vi "MEMR-Read Raw Data File (single traces).vi"(0 "Path":path=path "D:/Data/MEMR/Ken/SFMH41-MEMR-1.txt", 7 "index":i32, 9 "length":i32, 11 "error in":errorcluster) -> (8 "Array":dbl[][](array[numeric]), 15 "error out":errorcluster)   [LabVIEW 2020]
uses:
  PXI DAQ VIs/Utility VIs/Array Dimensions (2D).vi
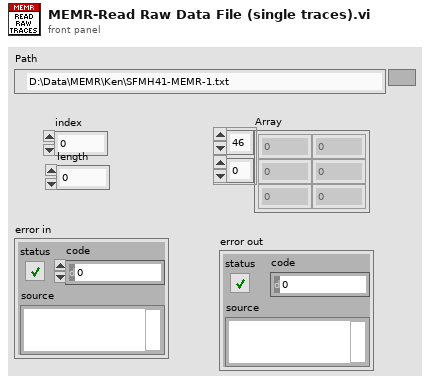
[diagram p1: front panel]
types:
  T1 = enum16{"open", "replace", "create", "open or create", "replace or create", "replace or create with confirmation"}
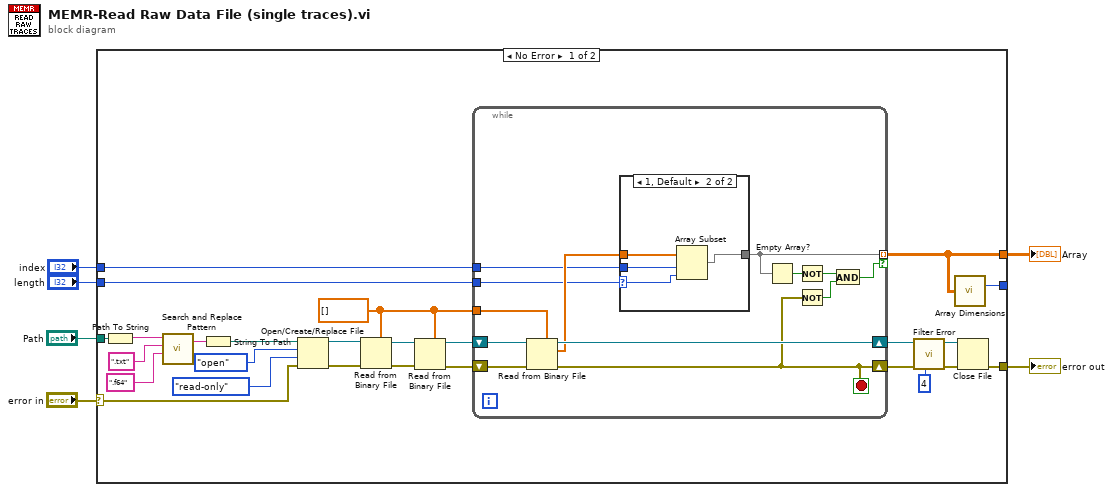
[diagram p0: block diagram]
diagram:
  n1 = case shown="No Error" "error in" {
    selector: "error in" -> [w13 w50]
    tunnel: "Path" -> [w14 _]
    tunnel: [w12 w50] -> w4
    tunnel: [w8 _] -> w3
    tunnel: "index" -> [w10 _]
    tunnel: "length" -> [w9 _]
    tunnel: [w7 _] -> _
    frame No Error {
      w11 = dbl[] []
      n2 = Path To String(path=w14) -> (string=w31:string)
      n3 = call <vilib>:"Search and Replace Pattern.vi"("string"=w31, "regular expression (\"\")"=".txt" ("regular expression (\"\")"), "replace string (\"\")"=".f64" ("replace string (\"\")")) -> ("result string"=w28:string)  [unwired: 2 in, 1 out]
      n4 = String To Path(string=w28) -> (path=w27:path)
      n5 = Open/Create/Replace File(file path (use dialog)=w27, error in=w13, operation (0:open)=T1."open", access (0:read/write)=enum16{"read/write", "read-only", "write-only"}."read-only") -> (refnum out=w23:refnum<file>, error out=w24:errorcluster)  [unwired: 2 in, 1 out]
      n6 = Read from Binary File(5:w11, 8:w24, 11:w23) -> (0:w22:errorcluster, 3:w21:refnum<file>)  [unwired: 3 in, 2 out]
      n7 = Read from Binary File(5:w11, 8:w22, 11:w21) -> (0:w19:errorcluster, 3:w20:refnum<file>)  [unwired: 3 in, 2 out]
      n8 = while {
        shift-right: [w42] -> w18
        shift-left: w20 -> [w44]
        shift-right: [w33] -> w17
        shift-left: w19 -> [w43]
        tunnel: [w35] -> w8 mode=indexing if=w34
        tunnel: w11 -> [w39]
        tunnel: w10 -> [w37]
        tunnel: w9 -> [w36]
        stop <- w33 stop-if-true
        n9 = Read from Binary File(5:w39, 8:w43, 11:w44) -> (0:w33:errorcluster, 2:w38:dbl[], 3:w42:refnum<file>)  [unwired: 3 in, 1 out]
        n10 = case shown="1, Default" w36 {
          selector: w36 -> [_ w47]
          tunnel: w38 -> [w45 w49]
          tunnel: w37 -> [_ w48]
          tunnel: [w45 w46] -> w35
          frame 0 {
          }
          frame 1, Default {
            n11 = Array Subset(array=w49, index=w48, length=w47) -> (w46:dbl[])
          }
        }
        n12 = Empty Array?(array=w35) -> (empty?=w41:bool)
        n13 = Not(x=w41) -> (.not. x?=w40:bool)
        n14 = Not(x=w33) -> (.not. x?=w32:bool)
        n15 = And(x=w40, y=w32) -> (x .and. y?=w34:bool)
      }
      n16 = call "Filter Error.vi"("error in (no error)"=w17, "code to ignore"=4) -> ("error out"=w16:errorcluster)  [unwired: 9 in]
      n17 = call-poly "Array Dimensions.vi"("2D Array"=w8) -> ("# rows"=w7:i32)  [unwired: 13 in, 1 out]
      n18 = Close File(refnum=w18, error in=w16) -> (error out=w12:errorcluster)  [unwired: 1 out]
    }
    frame Error {
    }
  }
  "error out" <- w4
  "Array" <- w3
